vi "CPP_Aeroprobe_TimeSeries.vi"() -> (5 "Plug in titles":string[](array[string]), 7 "Plug in values":string[](array[string]))   [LabVIEW 2012]
uses:
  Globals/Meas_global.vi
  <vilib>/Analysis/NI_AALBase.lvlib
panel:
  in  "Calibration Folder Path":path=path "I:/5HoleProbe"
  in  "Correction File Path":path=path "M:/Preferences/Rig_Setups/All_Rigs/TubingCompensation/5HPTubingCorrection12066.xls"
  in  "Apply Phase Correction?":bool=TRUE
  out "DataArray":dbl[](array[numeric])
  out "Zeroes":dbl[](array[numeric])
  out "Progress":dbl(slide) scale=-1.0..820.0
  in  "Old5HoleProbe?":bool
  # "!! 5-hole 1-5 must be connected to Channels 1-5 !!"
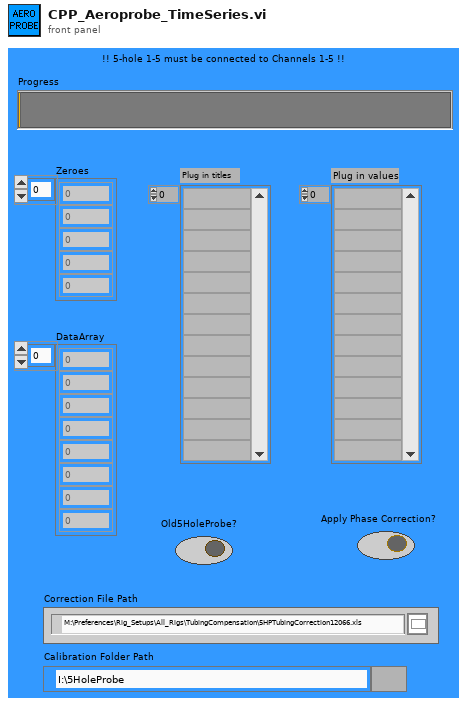
[diagram p1: front panel]
types:
  T1 = typedef "Analysis_info_cluster.ctl" = cluster{"Colour":u32, "Inst type":T2, "Inst name":string, "Symbol":string, "Code name":string, "Extra Info":string, "Inst Array":T3, "Extra Titles":string[], "Extra Values":string[], "U":dbl, "u^2":dbl, "u^3":dbl, "u^4":dbl, "Skew_u":dbl, "Kurt_u":dbl, "Sd Error in Mean":dbl, "% u'/U":dbl, "X":dbl, "Y":dbl, "Z":dbl, "Timescale integral to 25%":dbl, "Sd Error in Variance":dbl, "Calib File":path, "Calib Constants":dbl[], "Output Position":bool, "Full Stats":bool, "Av Sampling Rate":dbl, "Av No of Samples":dbl, "Total Meas Time (s)":dbl, "ADAM Ch Name":string}
  T2 = typedef "Inst_type.ctl" = enum16{"Propeller anemometer", "Raw voltage", "Pressure Transducer", "Pitot-static tube", "Preston tube", "Hot wire", "Cross wire 1", "Cross wire 2", "Generic Linear", "Generic Polynomial", "Generic BackPoly", "Fast FID", "Thermocouple", "Cold wire", "Pulsed Wire", "LDA Vel", "LDA Tran time", "LDA Arr time"}
  T3 = typedef "Instrument_Array.ctl" = enum16{"PWA", "LDA", "Analogue"}
  T4 = cluster{"Analysis Info cluster[0]":T1, "Analysis Info cluster[1]":T1, "Analysis Info cluster[2]":T1, "Analysis Info cluster[3]":T1, "Analysis Info cluster[4]":T1, "Analysis Info cluster[5]":T1, "Analysis Info cluster[6]":T1}
  T5 = typedef "Time_Trace_Cluster.ctl" = cluster{"Weighting":dbl[], "Time (s)":dbl[], "Voltage":dbl[], "Eng Values":dbl[]}
  T6 = cluster{"[0]":dbl, "[1]":dbl, "[2]":dbl, "[3]":dbl, "[4]":dbl}
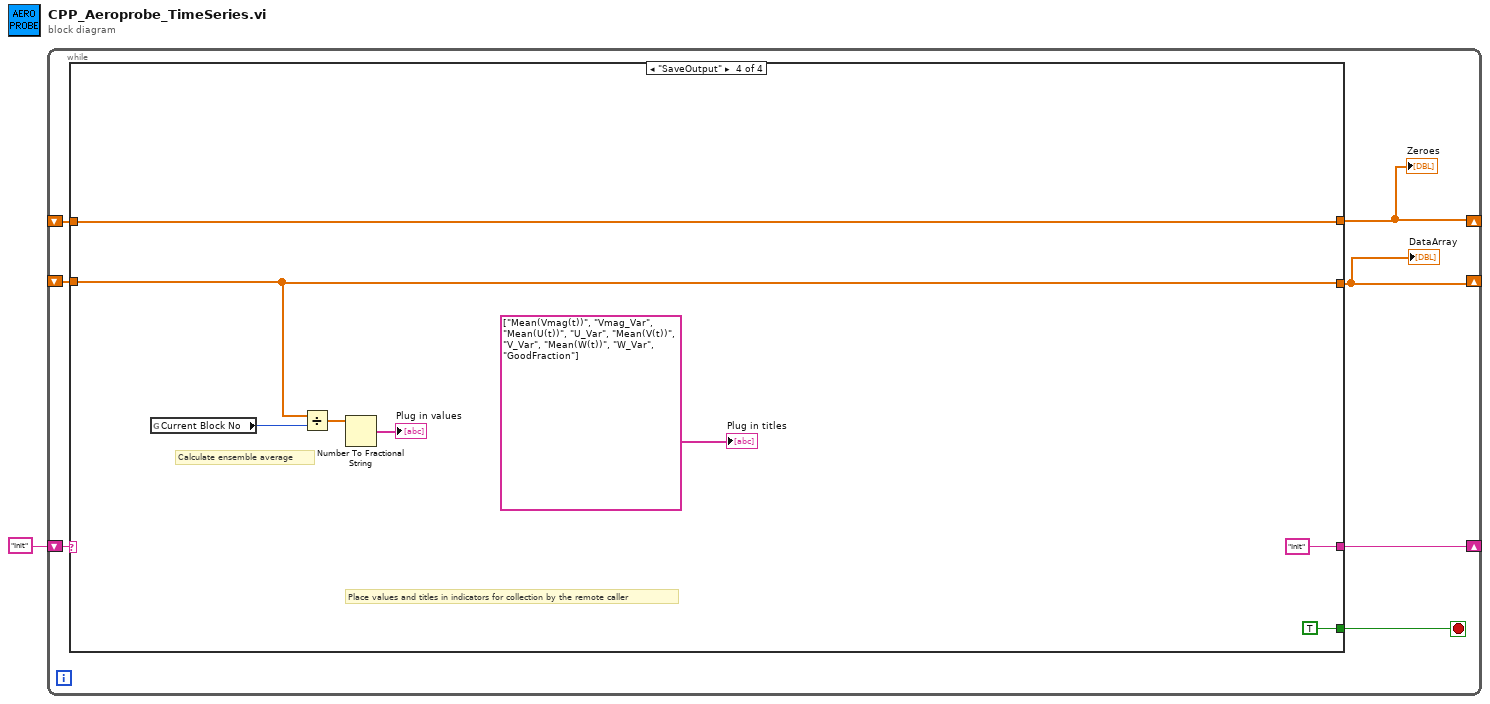
[diagram p0: block diagram]
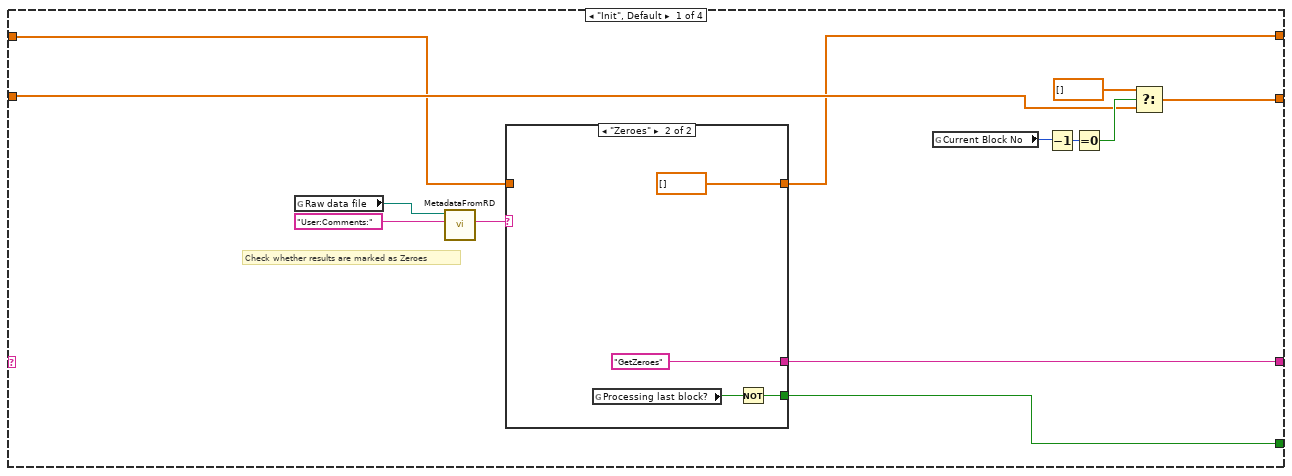
[diagram p2: hidden frame]
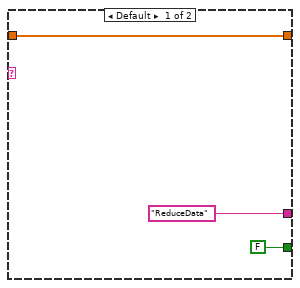
[diagram p3: hidden frame]
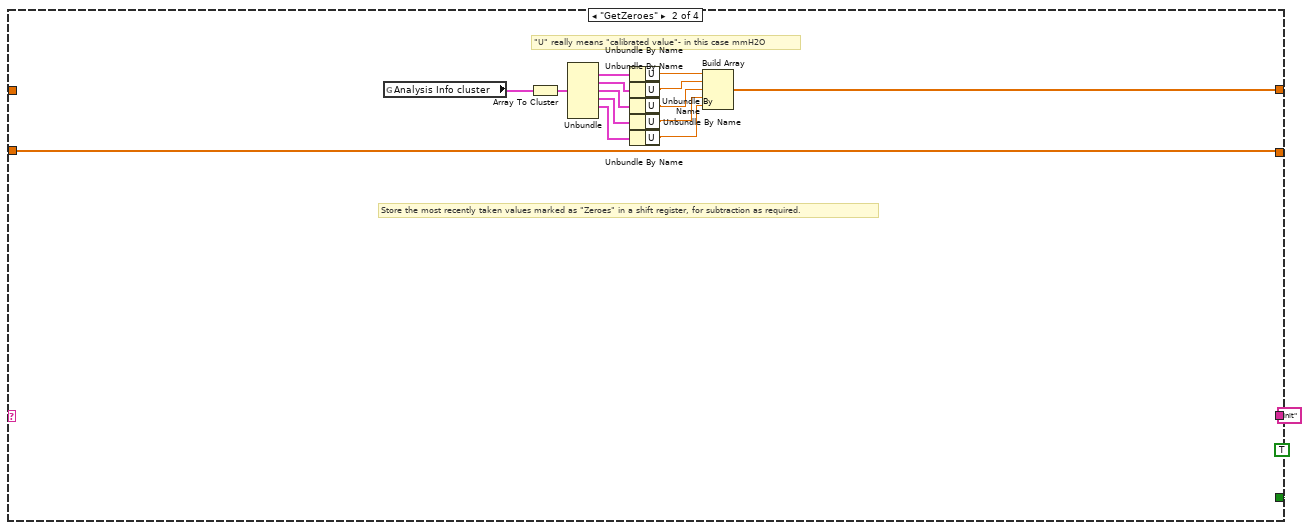
[diagram p4: hidden frame]
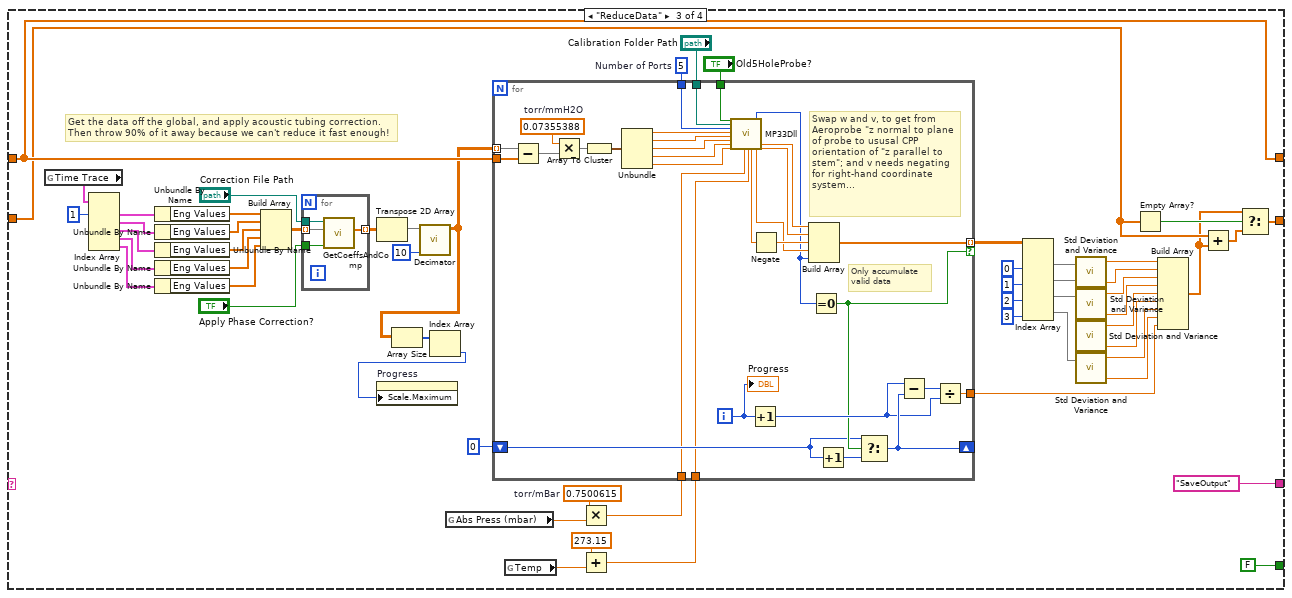
[diagram p5: hidden frame]
diagram:
  n1 = while {
    shift-right: [w7] -> _
    shift-left: "Init" -> [w8]
    shift-right: [w6] -> _
    shift-left: _ -> [w5]
    shift-right: [w4] -> _
    shift-left: _ -> [w3]
    stop <- w2 stop-if-true
    n2 = case shown="\"SaveOutput\"" w8 {
      tunnel: [w21 "Init" "SaveOutput" "Init"] -> w7
      tunnel: [w11 w31 w100 w144] -> w6
      tunnel: w5 -> [w12 _ w100 w144]
      tunnel: [w14 w29 w69 w138] -> w4
      tunnel: w3 -> [w15 w29 w72 w138]
      tunnel: [w17 TRUE FALSE TRUE] -> w2
      frame "Init", Default {
        # "Check whether results are marked as Zeroes"
        n3 = global read "Meas_global.vi" "Raw data file"() -> (w20:path)
        n4 = call "MetadataFromRD.vi"("ChannelName"="User:Comments:", "Raw data file"=w20) -> ("ValueString"=w18:string)  [unwired: 8 in, 1 out]
        n5 = case shown="\"Zeroes\"" w18 {
          tunnel: ["ReduceData" "GetZeroes"] -> w21
          tunnel: [FALSE w27] -> w17
          tunnel: w12 -> [w22 _]
          tunnel: [w22 dbl[] [] ("t")] -> w11
          frame Default {
          }
          frame "Zeroes" {
            n6 = global read "Meas_global.vi" "Processing last block?"() -> (w26:bool)
            n7 = Not(x=w26) -> (.not. x?=w27:bool)
          }
        }
        n8 = global read "Meas_global.vi" "Current Block No"() -> (w10:i32)
        n9 = Decrement(x=w10) -> (x-1=w9:i32)
        n10 = Equal To 0?(x=w9) -> (x = 0?=w16:bool)
        n11 = Select(t=dbl[] [], s=w16, f=w15) -> (s? t:f=w14:dbl[])
      }
      frame "GetZeroes" {
        # "Store the most recently taken values marked as \"Zeroes\" in a shift register, for subtraction as required."
        # "\"U\" really means \"calibrated value\"- in this case mmH2O"
        n12 = global read "Meas_global.vi" "Analysis Info cluster"() -> (w33:T1[])
        n13 = Array To Cluster(array=w33) -> (cluster=w39:T4)
        n14 = Unbundle(w39) -> ("Analysis Info cluster[1]"=w40:T1, "Analysis Info cluster[2]"=w41:T1, "Analysis Info cluster[3]"=w42:T1, "Analysis Info cluster[4]"=w43:T1, "Analysis Info cluster[5]"=w44:T1)  [unwired: 2 out]
        n15 = Unbundle By Name(w40) -> ("U"=w38:dbl)
        n16 = Unbundle By Name(w41) -> ("U"=w37:dbl)
        n17 = Unbundle By Name(w42) -> ("U"=w36:dbl)
        n18 = Unbundle By Name(w43) -> ("U"=w35:dbl)
        n19 = Unbundle By Name(w44) -> ("U"=w34:dbl)
        n20 = Build Array(w38, w37, w36, w35, w34) -> (w31:dbl[])
      }
      frame "ReduceData" {
        w46 = 0.7500615  # torr/mBar
        w52 = 5  # Number of Ports
        # "Get the data off the global, and apply acoustic tubing correction. \nThen throw 90% of it away because we can't reduce it fast enough!"
        n21 = global read "Meas_global.vi" "Time Trace"() -> (w82:T5[])
        n22 = Index Array(array=w82, index #1=1 ("index")) -> (element #1=w81:T5, element #2=w90:T5, element #3=w89:T5, element #4=w88:T5, element #5=w87:T5)  [unwired: 4 in]
        n23 = Unbundle By Name(w81) -> ("Eng Values"=w80:dbl[])
        n24 = Unbundle By Name(w90) -> ("Eng Values"=w86:dbl[])
        n25 = Unbundle By Name(w89) -> ("Eng Values"=w85:dbl[])
        n26 = Unbundle By Name(w88) -> ("Eng Values"=w84:dbl[])
        n27 = Unbundle By Name(w87) -> ("Eng Values"=w83:dbl[])
        n28 = Build Array(w80, w86, w85, w84, w83) -> (w62:dbl[][])
        n29 = for {
          tunnel: w62 -> [w105] mode=indexing
          tunnel: [w104] -> w59 mode=indexing
          tunnel: "Apply Phase Correction?" -> [w103]
          tunnel: "Correction File Path" -> [w102]
          n30 = call "GetCoeffsAndComp.vi"("Apply Phase Correction?"=w103, "mutedData"=w105, "TubingCorrectionFile (pre-set!)"=w102) -> ("boostedData"=w104:dbl[])  [unwired: 8 in]
        }
        n31 = Transpose 2D Array(2D array=w59) -> (transposed array=w58:dbl[][])
        n32 = call "Decimator.vi"("Divider"=10, "Array In"=w58) -> ("Array Out"=w56:dbl[][])  [unwired: 9 in]
        n33 = Array Size(array=w56) -> (size(s)=w55:i32[])
        n34 = Index Array(array=w55) -> (element=w54:i32)  [unwired: 1 in]
        n35 = property on="Progress" class="Slide (strict)"("Scale.Maximum"=w54) -> ()  [unwired: 2 in, 2 out]
        n36 = global read "Meas_global.vi" "Abs Press (mbar)"() -> (w47:dbl)
        n37 = global read "Meas_global.vi" "Temp"() -> (w50:dbl)
        n38 = Multiply(x=w46, y=w47) -> (x*y=w45:dbl)
        n39 = Add(x=273.15, y=w50) -> (x+y=w48:dbl)
        n40 = for {
          tunnel: w56 -> [w123] mode=indexing
          tunnel: w100 -> [w122]
          tunnel: [w121] -> w79 mode=indexing if=w113
          shift-right: [w117] -> _
          shift-left: 0 -> [w111]
          tunnel: [w114] -> w64
          tunnel: "Calibration Folder Path" -> [w110]
          tunnel: w52 -> [w109]
          tunnel: "Old5HoleProbe?" -> [w108]
          tunnel: w48 -> [w107]
          tunnel: w45 -> [w106]
          i -> [w119]
          w136 = 0.07355388  # torr/mmH2O
          # "Only accumulate\nvalid data"
          # "Swap w and v, to get from Aeroprobe \"z normal to plane of probe to ususal CPP orientation of \"z parallel to stem\"; and v needs negating for right-hand coordinate system..."
          n41 = Subtract(x=w123, y=w122) -> (x-y=w120:dbl[])
          n42 = Multiply(x=w136, y=w120) -> (x*y=w135:dbl[])
          n43 = Array To Cluster(array=w135) -> (cluster=w134:T6)
          n44 = Unbundle(w134) -> ("[0]"=w133:dbl, "[1]"=w132:dbl, "[2]"=w131:dbl, "[3]"=w130:dbl, "[4]"=w129:dbl)
          n45 = call "MP33Dll.vi"("Old5HoleProbe?"=w108, "Calibration Folder Path"=w110, "Number of Ports"=w109, "P1 Torr"=w133, "P2 Torr"=w132, "P3 Torr"=w131, "P4 Torr"=w130, "P5 Torr"=w129, "Pref Torr"=w106, "TTot Kelvin"=w107) -> ("w m/s"=w126:dbl, "return type"=w118:i32, "v m/s"=w124:dbl, "VMagn m/s"=w128:dbl, "u  m/s"=w127:dbl)  [unwired: 7 in, 6 out]
          n46 = Increment(x=w119) -> (x+1=w115:i32)
          n47 = Negate(x=w126) -> (-x=w125:dbl)
          n48 = Build Array(w128, w127, w125, w124, w118) -> (w121:dbl[])
          n49 = Equal To 0?(x=w118) -> (x = 0?=w113:bool)
          n50 = Increment(x=w111) -> (x+1=w112:i32)
          n51 = Select(t=w111, s=w113, f=w112) -> (s? t:f=w117:i32)
          n52 = Subtract(x=w115, y=w117) -> (x-y=w116:i32)
          n53 = Divide(x=w116, y=w115) -> (x/y=w114:dbl)
          "Progress" <- w119
        }
        n54 = Index Array(array=w79, index (col) #1=0 ("disabled index (col)"), index (col) #2=1 ("index (col)"), index (col) #3=2 ("index (col)"), index (col) #4=3 ("index (col)")) -> (element #1=w99:dbl[], element #2=w98:dbl[], element #3=w97:dbl[], element #4=w96:dbl[])  [unwired: 4 in]
        n55 = call <vilib>:"Std Deviation and Variance.vi"("X"=w99) -> ("mean"=w95:dbl, "variance"=w68:dbl)  [unwired: 1 in, 1 out]
        n56 = call <vilib>:"Std Deviation and Variance.vi"("X"=w98) -> ("mean"=w94:dbl, "variance"=w67:dbl)  [unwired: 1 in, 1 out]
        n57 = call <vilib>:"Std Deviation and Variance.vi"("X"=w97) -> ("mean"=w93:dbl, "variance"=w66:dbl)  [unwired: 1 in, 1 out]
        n58 = call <vilib>:"Std Deviation and Variance.vi"("X"=w96) -> ("mean"=w92:dbl, "variance"=w65:dbl)  [unwired: 1 in, 1 out]
        n59 = Empty Array?(array=w72) -> (empty?=w71:bool)
        n60 = Build Array(w95, w68, w94, w67, w93, w66, w92, w65, w64) -> (w63:dbl[])
        n61 = Add(x=w72, y=w63) -> (x+y=w70:dbl[])
        n62 = Select(t=w63, s=w71, f=w70) -> (s? t:f=w69:dbl[])
      }
      frame "SaveOutput" {
        # "Place values and titles in indicators for collection by the remote caller"
        # "Calculate ensemble average"
        n63 = global read "Meas_global.vi" "Current Block No"() -> (w139:i32)
        n64 = Divide(x=w138, y=w139) -> (x/y=w137:dbl[])
        n65 = Number To Fractional String(number=w137) -> (F-format string=→"Plug in values":string[])  [unwired: 3 in]
        "Plug in titles" <- string[] ["Mean(Vmag(t))", "Vmag_Var", "Mean(U(t))", "U_Var", "Mean(V(t))", "V_Var", "Mean(W(t))", "W_Var", "GoodFraction"] ("Plug in titles")
      }
    }
    "Zeroes" <- w6
    "DataArray" <- w4
  }
